vi "Get Async Plugins.vi"(11 "Framework in":refnum<class "Framework.lvclass">) -> (2 "Async Plugins":refnum<class "Plugin.lvclass">[](array[class]), 3 "Framework out":refnum<class "Framework.lvclass">)   [LabVIEW 2017, in "DSF Core.lvlib" / "Framework.lvclass"]
uses:
  Framework.lvclass
  Plugin/Plugin.lvclass
  Framework.lvclass/Framework.ctl
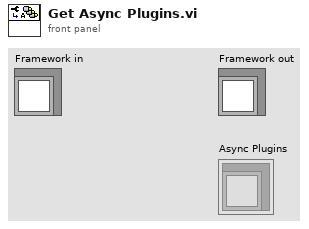
[diagram p1: front panel]
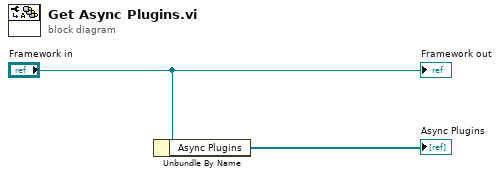
[diagram p0: block diagram]
diagram:
  n1 = Unbundle By Name("Framework in") -> ("Async Plugins"=→"Async Plugins":refnum<class "Plugin.lvclass">[])
  "Framework out" <- "Framework in"
